vi "Parse CSV.vi"(10 "End of Header":string="--\n", 11 "file path (use dialog)":path) -> (1 "Numeric Array":dbl[][](array[numeric]), 2 "Header":string, 3 "text":string)   [LabVIEW 2020]
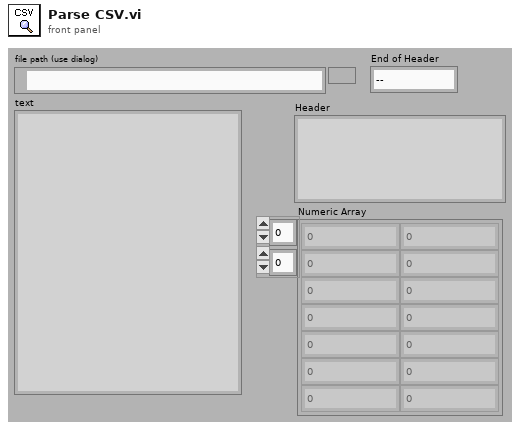
[diagram p1: front panel]
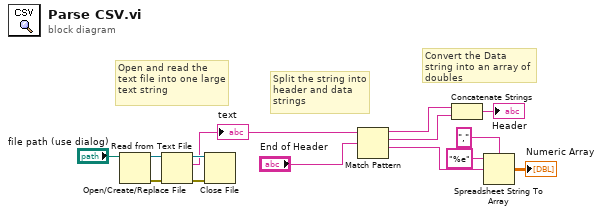
[diagram p0: block diagram]
diagram:
  # "Convert the Data string into an array of doubles"
  # "Split the string into header and data strings"
  # "Open and read the text file into one large text string"
  n1 = Open/Create/Replace File(file path (use dialog)="file path (use dialog)") -> (refnum out=w13:refnum<file>, error out=w12:errorcluster)  [unwired: 5 in, 1 out]
  n2 = Read from Text File(file (use dialog)=w13, error in=w12) -> (refnum out=w11:refnum<file>, text=w9:string, error out=w10:errorcluster)  [unwired: 2 in, 1 out]
  "text" <- w9
  n3 = Close File(refnum=w11, error in=w10) -> ()  [unwired: 2 out]
  n4 = Match Pattern(string=w9, regular expression="End of Header") -> (before substring=w3:string, match substring=w2:string, after substring=w7:string)  [unwired: 1 in, 1 out]
  n5 = Concatenate Strings(w3, w2) -> (→"Header":string)
  n6 = Spreadsheet String To Array(delimiter (Tab)=",", format string="%e", spreadsheet string=w7) -> (array=→"Numeric Array":dbl[][])  [unwired: 1 in]
